vi "Req_Driver.vi"(0 "URL":string, 2 "Output File":path=path "", 5 "Buffer":string, 11 "Error In":errorcluster, 12 "Timeout":i32=10000, 13 "Operation":T1) -> (4 "Headers":string, 6 "Body":string, 15 "Error Out":errorcluster)   [LabVIEW 2020]
doc: "This VI helps to make the REST API request with ease. This has all the four Get, Post, Put and delete request to be done."
uses:
  Typedef's/Request_Operations.ctl
  <vilib>/httpClient/POSTBuffer.vi
  <vilib>/httpClient/PUTBuffer.vi
  <vilib>/httpClient/LabVIEWHTTPClient.lvlib
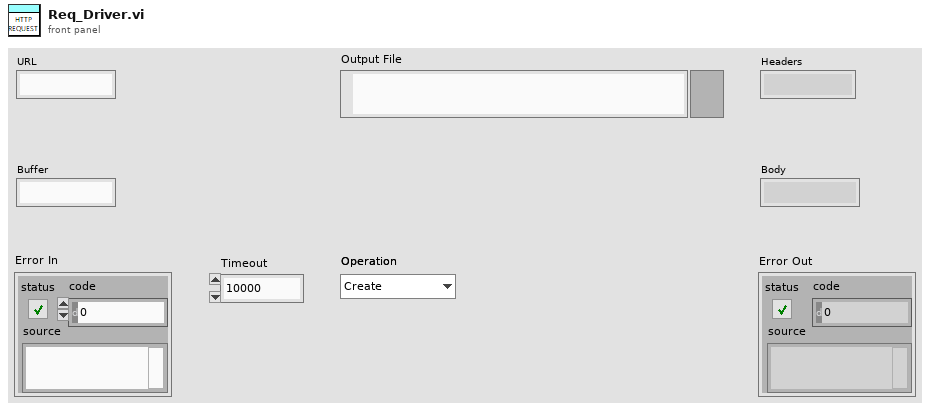
[diagram p1: front panel]
types:
  T1 = typedef "Request_Operations.ctl" = enum16{"Create", "Get", "Post", "Put", "Delete", "Destroy"}
  T2 = typedef "LabVIEWHTTPClient.lvlib/ClientHandle.ctl" = refnum<k1>
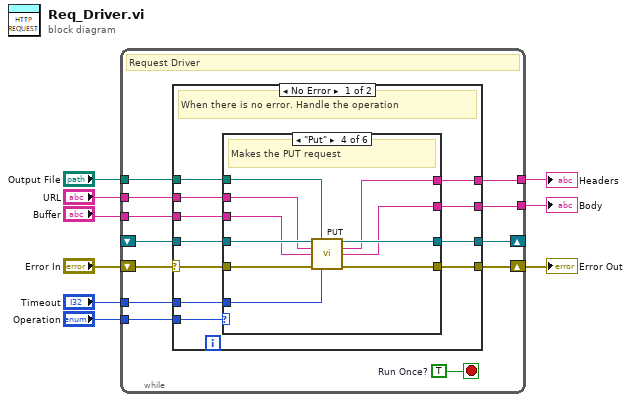
[diagram p0: block diagram]
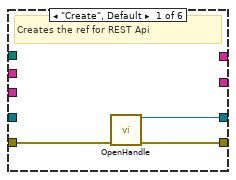
[diagram p2: hidden frame]
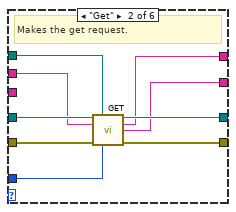
[diagram p3: hidden frame]
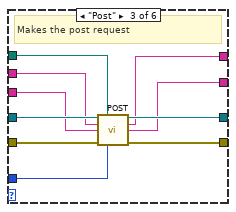
[diagram p4: hidden frame]
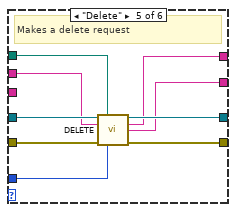
[diagram p5: hidden frame]
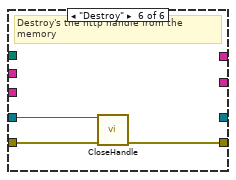
[diagram p6: hidden frame]
diagram:
  n1 = while {
    tunnel: "Operation" -> [w20]
    shift-right: [w18] -> w7
    shift-left: "Error In" -> [w19]
    shift-right: [w17] -> _
    shift-left: _ -> [w16]
    tunnel: "Timeout" -> [w15]
    tunnel: "URL" -> [w14]
    tunnel: "Output File" -> [w13]
    tunnel: [w12] -> w3
    tunnel: [w11] -> w2
    tunnel: "Buffer" -> [w10]
    stop <- w21 stop-if-true
    w21 = TRUE  # Run Once?
    # "Request Driver"
    n2 = case shown="No Error" w19 {
      selector: w19 -> [w31 w78]
      tunnel: w20 -> [w32 _]
      tunnel: [w30 w78] -> w18
      tunnel: [w29 w77] -> w17
      tunnel: w16 -> [w28 w77]
      tunnel: w15 -> [w27 _]
      tunnel: w14 -> [w26 _]
      tunnel: w13 -> [w25 _]
      tunnel: [w24 _] -> w12
      tunnel: [w23 _] -> w11
      tunnel: w10 -> [w22 _]
      frame No Error {
        # "When there is no error. Handle the operation"
        n3 = case shown="\"Put\"" w32 {
          tunnel: w31 -> [w35 w44 w54 w64 w73 w76]
          tunnel: [w34 w43 w53 w63 w72 w75] -> w30
          tunnel: [w33 w41 w51 w61 w70 _] -> w29
          tunnel: w28 -> [_ w42 w52 w62 w71 w74]
          tunnel: w27 -> [_ w40 w45 w55 w67 _]
          tunnel: w26 -> [_ w39 w49 w59 w68 _]
          tunnel: w25 -> [_ w38 w50 w60 w69 _]
          tunnel: [_ w37 w46 w57 w65 _] -> w24
          tunnel: [_ w36 w47 w56 w66 _] -> w23
          tunnel: w22 -> [_ _ w48 w58 _ _]
          frame "Create", Default {
            # "Creates the ref for REST Api"
            n4 = call <vilib>:"OpenHandle.vi"("error in (no error)"=w35) -> ("client handle out"=w33:T2, "error out"=w34:errorcluster)  [unwired: 13 in]
          }
          frame "Get" {
            # "Makes the get request."
            n5 = call <vilib>:"GET.vi"("client handle"=w42, "output file"=w38, "url"=w39, "error in (no error)"=w44, "timeout (10000)"=w40) -> ("client handle out"=w41:T2, "headers"=w37:string, "body"=w36:string, "error out"=w43:errorcluster)  [unwired: 7 in]
          }
          frame "Post" {
            # "Makes the post request"
            n6 = call-poly <vilib>:"POST.vi"("client handle"=w52, "output file"=w50, "url"=w49, "buffer"=w48, "error in (no error)"=w54, "timeout (10000)"=w45) -> ("client handle out"=w51:T2, "headers"=w46:string, "body"=w47:string, "error out"=w53:errorcluster)  [unwired: 6 in]
          }
          frame "Put" {
            # "Makes the PUT request"
            n7 = call-poly <vilib>:"PUT.vi"("client handle"=w62, "output file"=w60, "url"=w59, "buffer"=w58, "error in (no error)"=w64, "timeout (10000)"=w55) -> ("client handle out"=w61:T2, "headers"=w57:string, "body"=w56:string, "error out"=w63:errorcluster)  [unwired: 6 in]
          }
          frame "Delete" {
            # "Makes a delete request"
            n8 = call <vilib>:"DELETE.vi"("client handle"=w71, "output file"=w69, "url"=w68, "error in (no error)"=w73, "timeout (10000)"=w67) -> ("client handle out"=w70:T2, "headers"=w65:string, "body"=w66:string, "error out"=w72:errorcluster)  [unwired: 7 in]
          }
          frame "Destroy" {
            # "Destroy's the http handle from the memory"
            n9 = call <vilib>:"CloseHandle.vi"("client handle"=w74, "error in (no error)"=w76) -> ("error out"=w75:errorcluster)  [unwired: 13 in]
          }
        }
      }
      frame Error {
        # "when there is error. Do nothing"
      }
    }
  }
  "Error Out" <- w7
  "Headers" <- w3
  "Body" <- w2
